vi "InsertIntoCircularBuffer-Wfms.vi"(8 "NewElements":waveform(dbl)[](array[waveform]), 10 "StartIndex":dbl, 11 "Buffer":waveform(dbl)[](array[waveform])) -> (1 "New Start Index":dbl, 2 "UpdatedBuffer":waveform(dbl)[](array[waveform]))   [LabVIEW 2016]
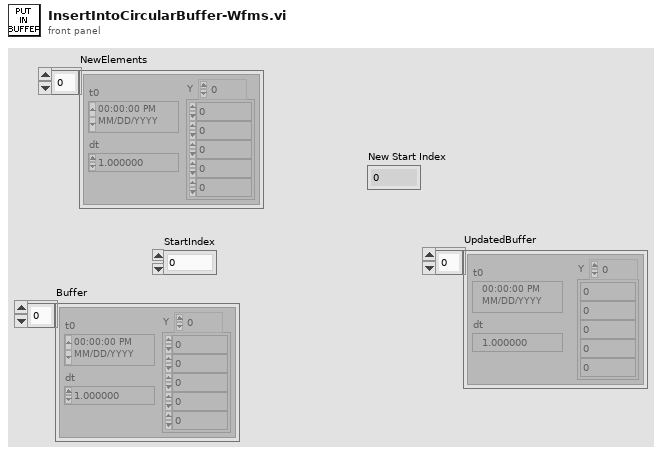
[diagram p1: front panel]
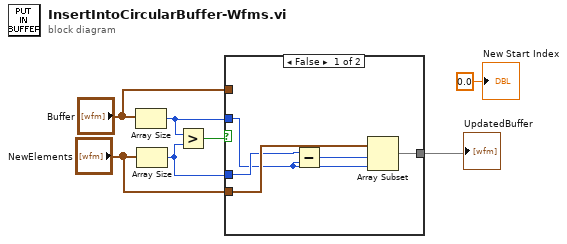
[diagram p0: block diagram]
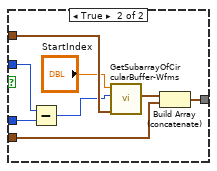
[diagram p2: hidden frame]
diagram:
  n1 = Array Size(array="Buffer") -> (size(s)=w6:i32)
  n2 = Array Size(array="NewElements") -> (size(s)=w5:i32)
  n3 = Greater?(x=w6, y=w5) -> (0:w7:bool)
  n4 = case shown="False" w7 {
    tunnel: w6 -> [w10 w20]
    tunnel: w5 -> [w11 w19]
    tunnel: "Buffer" -> [_ w16]
    tunnel: "NewElements" -> [w12 w18]
    tunnel: [w8 w13] -> w1
    frame False {
      n5 = Subtract(x=w11, y=w10) -> (x-y=w9:i32)
      n6 = Array Subset(array=w12, index=w9, length=w10) -> (w8:waveform(dbl)[])
    }
    frame True {
      n7 = Subtract(x=w20, y=w19) -> (x-y=w15:i32)
      n8 = call "GetSubarrayOfCircularBuffer-Wfms.vi"("buffer"=w16, "subset size"=w15, "start index"="StartIndex") -> ("subarray"=w17:waveform(dbl)[])  [unwired: 8 in]
      n9 = Build Array (concatenate)(w17, w18) -> (w13:waveform(dbl)[])
    }
  }
  "UpdatedBuffer" <- w1
  "New Start Index" <- 0.0 ("New Start Index")
